vi "GenericConfigureDrive.vi"(0 "Address":u8, 1 "Port Name":string, 2 "Channel Properties In":T1={"Channel Name"="", "Vel. Default"=5.0, "Acc. Default"=5.0, "Vel. Max"=5.0, "Vel. Min"=5.0, "Acc. Max"=5.0, "Acc. Min"=5.0, "Pulses/unit"=0.0, "Address"=0, "Pulse Offset"=0, "Pos Tolerance"=0.0, "Pulses/rev"=0.0, "Backlash/Eng units"=0.0, "Current Pos"=0.0, "Ch Status"=enum."Active", "Port Name"="", "Axis Transform mode"="", "Metadata Ch Name"="", "Type"=enum."MCode", "De Power Motor"=enum."FALSE", "ConfigString"=""} {"Current Pos" format="%.2f"; "Backlash/Eng units" format="%.2f"; "Pulses/rev" format="%.2f"; "Pos Tolerance" format="%.2f"; "Pulses/unit" format="%.2f"; "Acc. Min" format="%.2f"; "Acc. Max" format="%.2f"; "Vel. Min" format="%.2f"; "Vel. Max" format="%.2f"; "Acc. Default" format="%.2f"; "Vel. Default" format="%.2f"}, 3 "Channel Name":string) -> (8 "Good Echo":bool)   [LabVIEW 2022 SP3]
uses:
  ~subVIs/DriveProperties.ctl
  ~subVIs/Traverse Type.ctl
  Dynamixel/Sub Vis/Dynamixel Commands.ctl
  Dynamixel/Sub Vis/Dynamixel Global.vi
  Anemometry/Anemometry Sub Vis/Globals/Constants_global.vi
panel:
  out "Function Return":u32[](array[numeric])
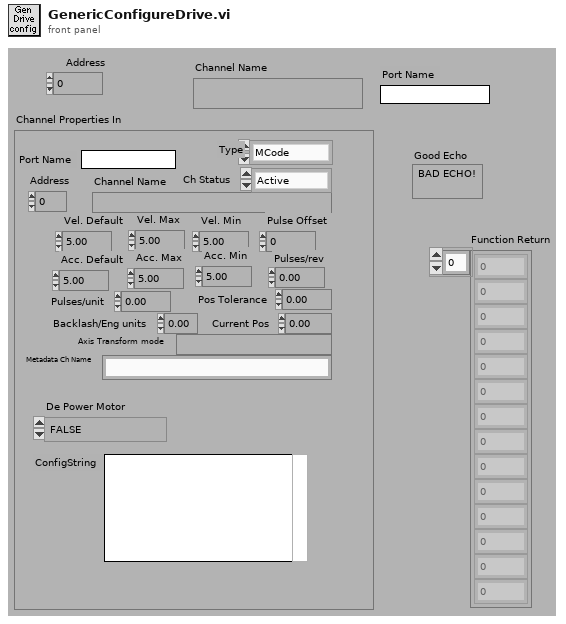
[diagram p1: front panel]
types:
  T1 = typedef "DriveProperties.ctl" = cluster{"Channel Name":string, "Vel. Default":sgl, "Acc. Default":sgl, "Vel. Max":sgl, "Vel. Min":sgl, "Acc. Max":sgl, "Acc. Min":sgl, "Pulses/unit":sgl, "Address":u8, "Pulse Offset":i32, "Pos Tolerance":sgl, "Pulses/rev":sgl, "Backlash/Eng units":sgl, "Current Pos":sgl, "Ch Status":enum16{"Active", "Offline", "Simulate"}, "Port Name":string, "Axis Transform mode":string, "Metadata Ch Name":string, "Type":T2, "De Power Motor":enum16{"TRUE", "FALSE"}, "ConfigString":string}
  T2 = typedef "Traverse Type.ctl" = enum16{"MCode", "Dynamixel"}
  T3 = typedef "Dynamixel Commands.ctl" = enum16{"Torque Enable", "Present Position", "Threshold", "Max Position Limit", "Acceleration Profile", "Velocity Profile", "Goal Position", "Position Proportional Gain", "Position Integral Gain", "Position Differential Gain ", "Shutdown", "Write Operating Mode", "Read Operating Mode"}
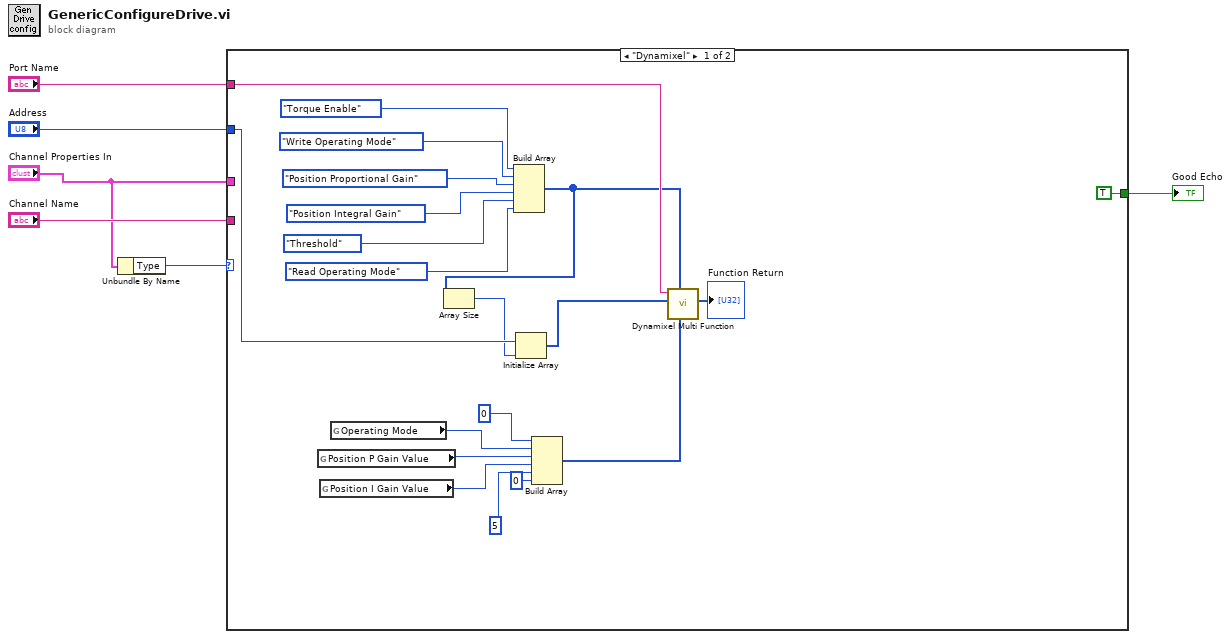
[diagram p0: block diagram]
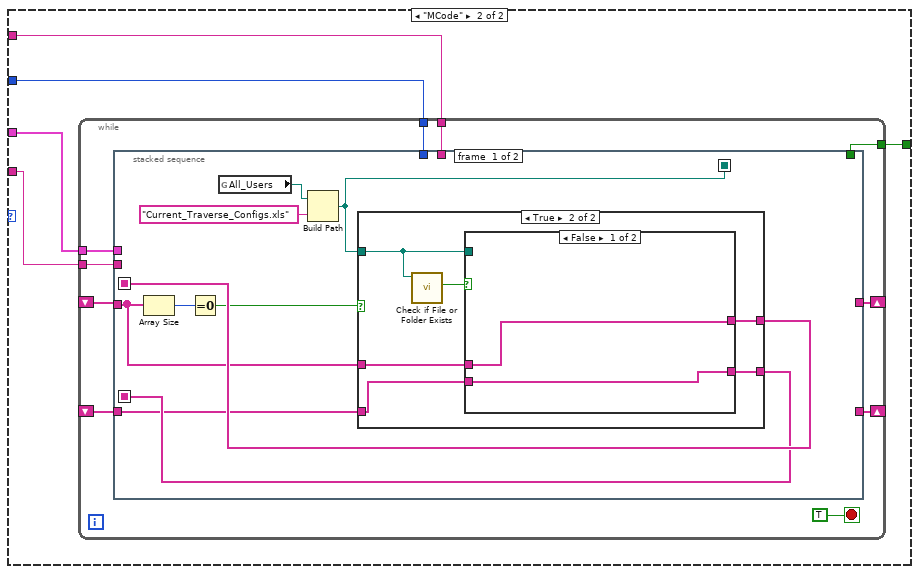
[diagram p2: hidden frame]
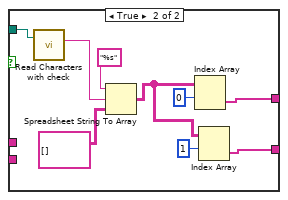
[diagram p4: hidden frame]
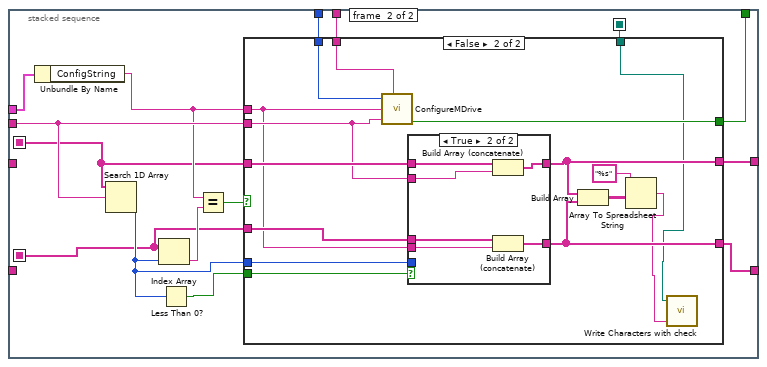
[diagram p5: hidden frame]
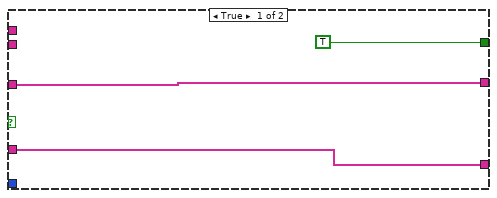
[diagram p6: hidden frame]
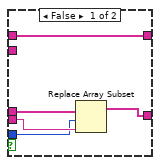
[diagram p7: hidden frame]
diagram:
  n1 = Unbundle By Name("Channel Properties In") -> ("Type"=w2:T2)
  n2 = case shown="\"Dynamixel\"" w2 {
    tunnel: "Address" -> [w24 w31]
    tunnel: "Channel Properties In" -> [_ w27]
    tunnel: "Port Name" -> [w25 w30]
    tunnel: "Channel Name" -> [_ w29]
    tunnel: [TRUE ("Good Echo") w28] -> w3
    frame "Dynamixel" {
      n3 = global read "Dynamixel Global.vi" "Position P Gain Value"() -> (w21:u32)
      n4 = global read "Dynamixel Global.vi" "Position I Gain Value"() -> (w11:u32)
      n5 = global read "Dynamixel Global.vi" "Operating Mode"() -> (w23:u8)
      n6 = Build Array(Dynamixel_Commands."Torque Enable" ("Function"), Dynamixel_Commands."Write Operating Mode" ("Function"), Dynamixel_Commands."Position Proportional Gain" ("Function"), Dynamixel_Commands."Position Integral Gain" ("Function"), Dynamixel_Commands."Threshold" ("Function"), Dynamixel_Commands."Read Operating Mode" ("Function")) -> (w18:T3[])
      n7 = Array Size(array=w18) -> (size(s)=w17:i32)
      n8 = Initialize Array(w24, w17) -> (w16:u8[])
      n9 = Build Array(u32 0 ("element"), w23, w21, w11, u32 5 ("element"), u32 0 ("element")) -> (w15:u32[])
      n10 = call "Dynamixel Multi Function.vi"("Data Array"=w15, "Function Array"=w18, "Motor ID"=w16, "Com port"=w25) -> ("Function Return"=→"Function Return":u32[])  [unwired: 6 in, 1 out]
    }
    frame "MCode" {
      n11 = while {
        tunnel: w31 -> [w41]
        tunnel: w30 -> [w40]
        tunnel: w29 -> [w35]
        tunnel: [w39] -> w28
        tunnel: w27 -> [w33]
        shift-right: [w38] -> _
        shift-left: _ -> [w34]
        shift-right: [w36] -> _
        shift-left: _ -> [w32]
        stop <- TRUE stop-if-true
        n12 = stacked-sequence {
          seq-local: [w46 _] -> [_ w71]
          seq-local: [w45 _] -> [_ w70]
          seq-local: [w47 _] -> [_ w72]
          tunnel: w41 -> [_ w84]
          tunnel: w40 -> [_ w83]
          tunnel: [_ w82] -> w39
          tunnel: [_ w81] -> w38
          tunnel: [_ w80] -> w36
          tunnel: w35 -> [_ w79]
          tunnel: w34 -> [w43 _]
          tunnel: w33 -> [_ w74]
          tunnel: w32 -> [w44 _]
          frame #0 {
            n13 = Array Size(array=w44) -> (size(s)=w50:i32)
            n14 = Equal To 0?(x=w50) -> (x = 0?=w42:bool)
            n15 = global read "Constants_global.vi" "All_Users"() -> (w49:path)
            n16 = Build Path(base path=w49, name or relative path="Current_Traverse_Configs.xls") -> (appended path=w47:path)
            n17 = case shown="True" w42 {
              tunnel: w47 -> [_ w56]
              tunnel: [w52 w58] -> w46
              tunnel: [w51 w57] -> w45
              tunnel: w44 -> [w52 w54]
              tunnel: w43 -> [w51 w53]
              frame False {
              }
              frame True {
                n18 = call <vilib>:"Check if File or Folder Exists.vi"("path"=w56) -> ("file or folder exists?"=w55:bool)  [unwired: 8 in, 2 out]
                n19 = case shown="False" w55 {
                  tunnel: [w60 w65] -> w58
                  tunnel: [w59 w64] -> w57
                  tunnel: w56 -> [_ w62]
                  tunnel: w54 -> [w60 _]
                  tunnel: w53 -> [w59 _]
                  frame False {
                  }
                  frame True {
                    n20 = call "Read Characters with check.vi"("file (use dialog)"=w62) -> ("Read String"=w61:string)  [unwired: 1 in, 1 out]
                    n21 = Spreadsheet String To Array(format string="%s", spreadsheet string=w61, array type (2D Dbl)=string[][] []) -> (array=w66:string[][])  [unwired: 1 in]
                    n22 = Index Array(array=w66, index (row)=0) -> (element=w65:string[])  [unwired: 1 in]
                    n23 = Index Array(array=w66, index (row)=1) -> (element=w64:string[])  [unwired: 1 in]
                  }
                }
              }
            }
          }
          frame #1 {
            n24 = Unbundle By Name(w74) -> ("ConfigString"=w73:string)
            n25 = Search 1D Array(1D array=w71, element=w79) -> (index of element=w75:i32)  [unwired: 1 in]
            n26 = Index Array(array=w70, index=w75) -> (element=w78:string)
            n27 = Less Than 0?(x=w75) -> (x < 0?=w76:bool)
            n28 = Equal?(x=w73, y=w78) -> (x = y?=w77:bool)
            n29 = case shown="False" w77 {
              tunnel: w84 -> [_ w102]
              tunnel: w83 -> [_ w101]
              tunnel: w79 -> [_ w97]
              tunnel: [TRUE ("Good Echo") w100] -> w82
              tunnel: w73 -> [_ w94]
              tunnel: [w86 w92] -> w81
              tunnel: w70 -> [w86 w99]
              tunnel: w71 -> [w85 w98]
              tunnel: [w85 w93] -> w80
              tunnel: w76 -> [_ w96]
              tunnel: w75 -> [_ w95]
              tunnel: w72 -> [_ w89]
              frame True {
              }
              frame False {
                n30 = call "ConfigureMDrive.vi"("Address"=w102, "Port Name"=w101, "ConfigString"=w94, "Channel Name"=w97) -> ("Good Echo"=w100:bool)  [unwired: 4 out]
                n31 = case shown="True" w96 {
                  tunnel: [w103 w113] -> w92
                  tunnel: w99 -> [w107 w112]
                  tunnel: w98 -> [w104 w111]
                  tunnel: [w104 w110] -> w93
                  tunnel: w94 -> [w106 w109]
                  tunnel: w97 -> [_ w108]
                  tunnel: w95 -> [w105 _]
                  frame False {
                    n32 = Replace Array Subset(array=w107, new element=w106, index=w105) -> (w103:string[])
                  }
                  frame True {
                    n33 = Build Array (concatenate)(w111, w108) -> (w110:string[])
                    n34 = Build Array (concatenate)(w112, w109) -> (w113:string[])
                  }
                }
                n35 = Build Array(w93, w92) -> (w91:string[][])
                n36 = Array To Spreadsheet String(array=w91, 3:"%s" ("format string")) -> (spreadsheet string=w88:string)  [unwired: 1 in]
                n37 = call "Write Characters with check.vi"("String to Write"=w88, "file (use dialog)"=w89) -> ()  [unwired: 2 in, 1 out]
              }
            }
          }
        }
      }
    }
  }
  "Good Echo" <- w3
